vi "Custom Borders to PdfPCells.vi"(0 "PDF Report":T29(xcontrol), 7 "Custom Borders":T11={"Title Row Border"={"Line"={"Thickness"=1.0, "Color"=0}, "Column Borders [ ]"=[]}, "Datas Row Borders [ ]"=[]}, 9 "Cell [ ]":T7[](array[typedef]), 11 "error in (no error)":errorcluster, 12 "Title format":T2={"Font Ref"=refnum, "Leading"=18.0, "Horizontal Aligment"=enum."JUSTIFY", "Vertical Alignment"=enum."BOTTOM"}, 13 "Data Format":T2={"Font Ref"=refnum, "Leading"=18.0, "Horizontal Aligment"=enum."JUSTIFY", "Vertical Alignment"=enum."BOTTOM"}) -> (4 "PDF Report duplicate":T29(xcontrol), 6 "Datas Row Cells [ ]":T1, 10 "Title Row Cells":T6={"Cell Cluster"={"Font Ref"=refnum, "Leading"=18.0, "Horizontal Aligment"=enum."JUSTIFY", "Vertical Alignment"=enum."BOTTOM"}, "PdfPCell [ ]"=[]}, 15 "error out":errorcluster)   [LabVIEW 2012]
doc: "Version 1.0\nDeveloped by Jean-Marc Simard\nCopyright © 2010, Exaprom Inc.\nAll rights reserved.\nLicense: BSD\n\nWith iTextSharp 4.1.6 (http://itextsharp.sourceforge.net)\nunder Mozilla Public License Version 1.1\n(http://www.mozilla.org/MPL/MPL-1.1.html)"
uses:
  Controls/PDF Report Xcontrol/PDF Report.xctl
  Controls/Row Border Title.ctl
  Controls/Cell Border.ctl
  Controls/Row Borders [ ] Datas.ctl
  Controls/Cell Cluster.ctl
  C:/Users/MaxCorp/Documents/TopPerm - Base/DLL/itextsharp.dll
  DLL/itextsharp.dll
  Controls/Font size.ctl
  Controls/Texte alignement.ctl
  Controls/Cell Vertical alignment.ctl
  Controls/Cell Generic Format without Font.ctl
  Controls/Title Cells with refnum.ctl
  Controls/Row PdfPCell [ ] Datas.ctl
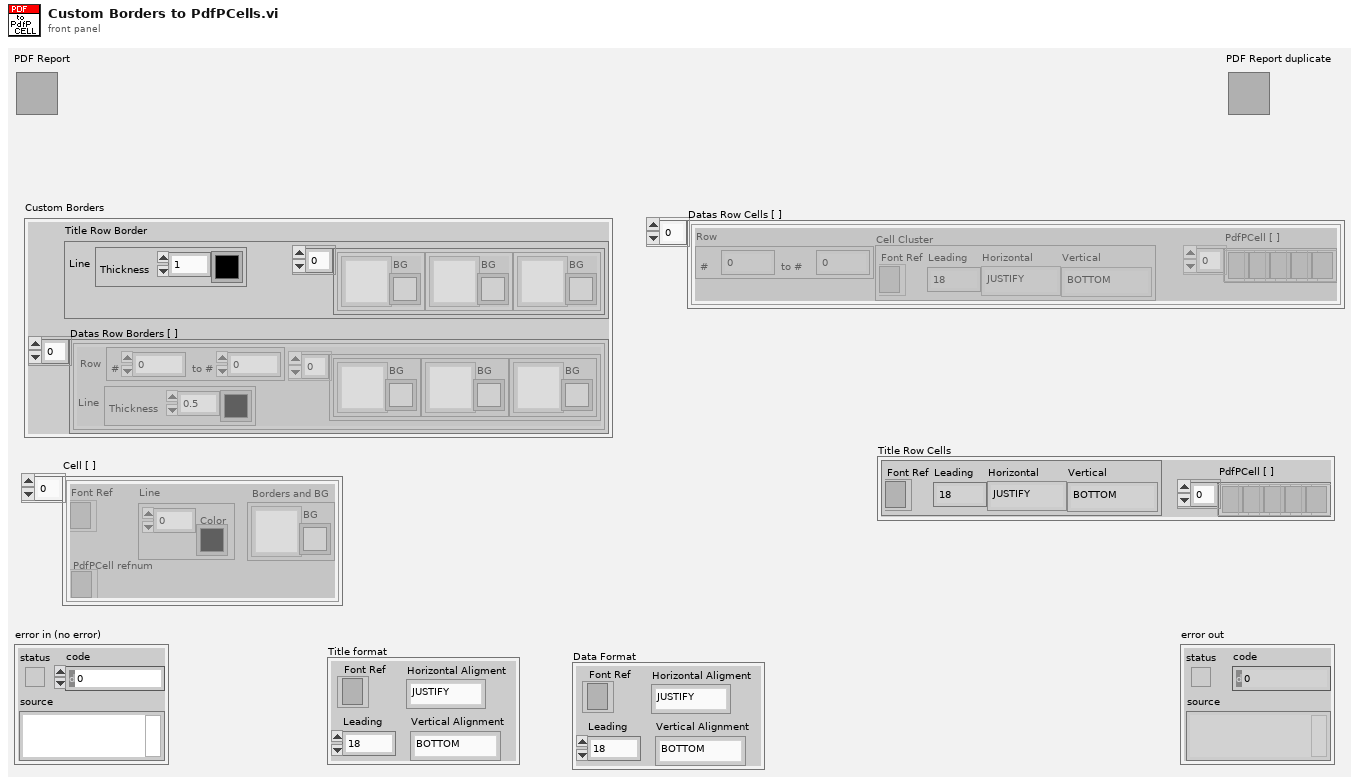
[diagram p1: front panel]
types:
  T1 = typedef "Row PdfPCell [ ] Datas.ctl" = cluster{"Row":cluster{"#":i16, "to #":i16}, "Cell Cluster":T2, "PdfPCell [ ]":refnum<k24>[]}[]
  T2 = typedef "Cell Cluster.ctl" = cluster{"Font Ref":refnum<k24>, "Leading":T3, "Horizontal Aligment":T4, "Vertical Alignment":T5}
  T3 = typedef "Font size.ctl" = sgl
  T4 = typedef "Texte alignement.ctl" = enum16{"Select", "CENTER", "JUSTIFY", "LEFT", "RIGHT"}
  T5 = typedef "Cell Vertical alignment.ctl" = enum16{"TOP", "MIDDLE", "BOTTOM"}
  T6 = typedef "Title Cells with refnum.ctl" = cluster{"Cell Cluster":T2, "PdfPCell [ ]":refnum<k24>[]}
  T7 = typedef "Cell Generic Format without Font.ctl" = cluster{"Font Ref":refnum<k24>, "Line":cluster{"Thickness":sgl, "Color":u32}, "Borders and BG":cluster{"Cell Border":T8, "BG":u32}, "PdfPCell refnum":refnum<k24>}
  T8 = typedef "Cell Border.ctl" = u16
  T9 = typedef "Row Border Title.ctl" = cluster{"Line":cluster{"Thickness":sgl, "Color":u32}, "Column Borders [ ]":cluster{"Cell Border":T8, "BG":u32}[]}
  T10 = typedef "Row Borders [ ] Datas.ctl" = cluster{"Row":cluster{"#":i16, "to #":i16}, "Line":cluster{"Thickness":sgl, "Color":u32}, "Column Borders [ ]":cluster{"Cell Border":T8, "BG":u32}[]}[]
  T11 = cluster{"Title Row Border":T9, "Datas Row Borders [ ]":T10}
  T12 = typedef "Font cluster.ctl" = cluster{"Name":string, "Size":T3, "Color":T13, "Style":cluster{"Bold":bool, "Italic":bool, "Underline":bool, "Strikeout":bool}}
  T13 = typedef "Font color.ctl" = u32
  T14 = typedef "Unit.ctl" = enum16{"inch", "mm"}
  T15 = typedef "Paragraphe cluster.ctl" = cluster{" Aligment":T4, "Line spacing":T16}
  T16 = typedef "Line spacing.ctl" = enum16{"Select", "1.0", "1.5", "2.0"}
  T17 = typedef "Page dimensions.ctl" = cluster{"Start at page":i32, "Orientation":T18, "widht":sgl, "height":sgl, "Margin left":sgl, "Margin right":sgl, "Margin top":sgl, "Margin bottom":sgl}
  T18 = typedef "Page Orientation.ctl" = enum16{"Portrait", "Landscape"}
  T19 = typedef "Image or Table Caption.ctl" = cluster{"Caption":string, "Separator":string, "Position":enum16{"Above", "Below"}}
  T20 = typedef "Header Footer [ ].ctl" = T21[]
  T21 = typedef "Header Footer cluster.ctl" = cluster{"Start page":i32, "Type":T22, "Alignment":T23, "Vertical Alignement":T5, "Image (%)":sgl, "Page #":T24, "Text":string, "Path":string, "Font":T12, "Font refnum":refnum<k24>, "Line":cluster{"Line":T25, "Thickness (points)":sgl, "Colour":T13}}
  T22 = typedef "Header Footer Type.ctl" = enum16{"Select", "Text", "Text + hyperlink", "Page number", "Image", "Image + hyperlink"}
  T23 = typedef "Header footer horiz alignment.ctl" = enum16{"Left", "Center", "Right"}
  T24 = typedef "Page number.ctl" = cluster{"Text 1":string, "Text 2":string, "Text 3":string}
  T25 = typedef "Header Footer Line.ctl" = enum16{"No line", "Horizontal line"}
  T26 = typedef "Watermark cluster2.ctl" = cluster{"Show? (F)":bool, "Type":enum16{"Image", "Text"}, "Opacity (%)":sgl, "Rotate(°)":sgl, "Position":cluster{"Position":T27, "X":sgl, "Y":sgl}, "Image path":path, "Scaled(%)":sgl, "Image refnum":refnum<k24>, "Text":string, "Font":cluster{"Name":string, "Size":T3, "Color":T13}, "Font refnum":refnum<k24>, "Alignment":T23, "Automatic":bool}
  T27 = typedef "Watermark Position.ctl" = enum16{"Absolute", "Center (page)", "Center (text section)"}
  T28 = typedef "System Fonts.ctl" = cluster{"Font name [ ]":string[], "Font and file names [ ]":cluster{"Font name":string, "File name":string}[]}
  T29 = cluster{"Document":refnum<k24>, "Writer":refnum<k24>, "Default Font":refnum<k24>, "Default Font cluster":T12, "Path":path, "Unit (default = mm)":T14, "Paragraphe cluster":T15, "Pages dimensions [ ]":T17[], "Captions":cluster{"Image":T19, "Image counter":u16, "Table":T19, "Table counter":u16, "Font":T12}, "Header":T20, "Footer":T20, "Watermark ":T26, "Actual VI name":string, "System Fonts":T28}
  T30 = cluster{"Row":cluster{"#":i16, "to #":i16}, "Cell Cluster":T2, "PdfPCell [ ]":refnum<k24>[]}
  T31 = cluster{"Row":cluster{"#":i16, "to #":i16}, "Cell Cluster":T2, "PdfPCell [ ]":refnum<k24>[]}[]
  T32 = cluster{"Font Ref":refnum<k24>, "Line":cluster{"Thickness":sgl, "Color":u32}, "Borders and BG":cluster{"Cell Border":T8, "BG":u32}}
  T33 = cluster{"Font Ref":refnum<k24>, "Line":cluster{"Thickness":sgl, "Color":u32}, "Cluster 2":cluster{"Cell Border":T8, "BG":u32}}
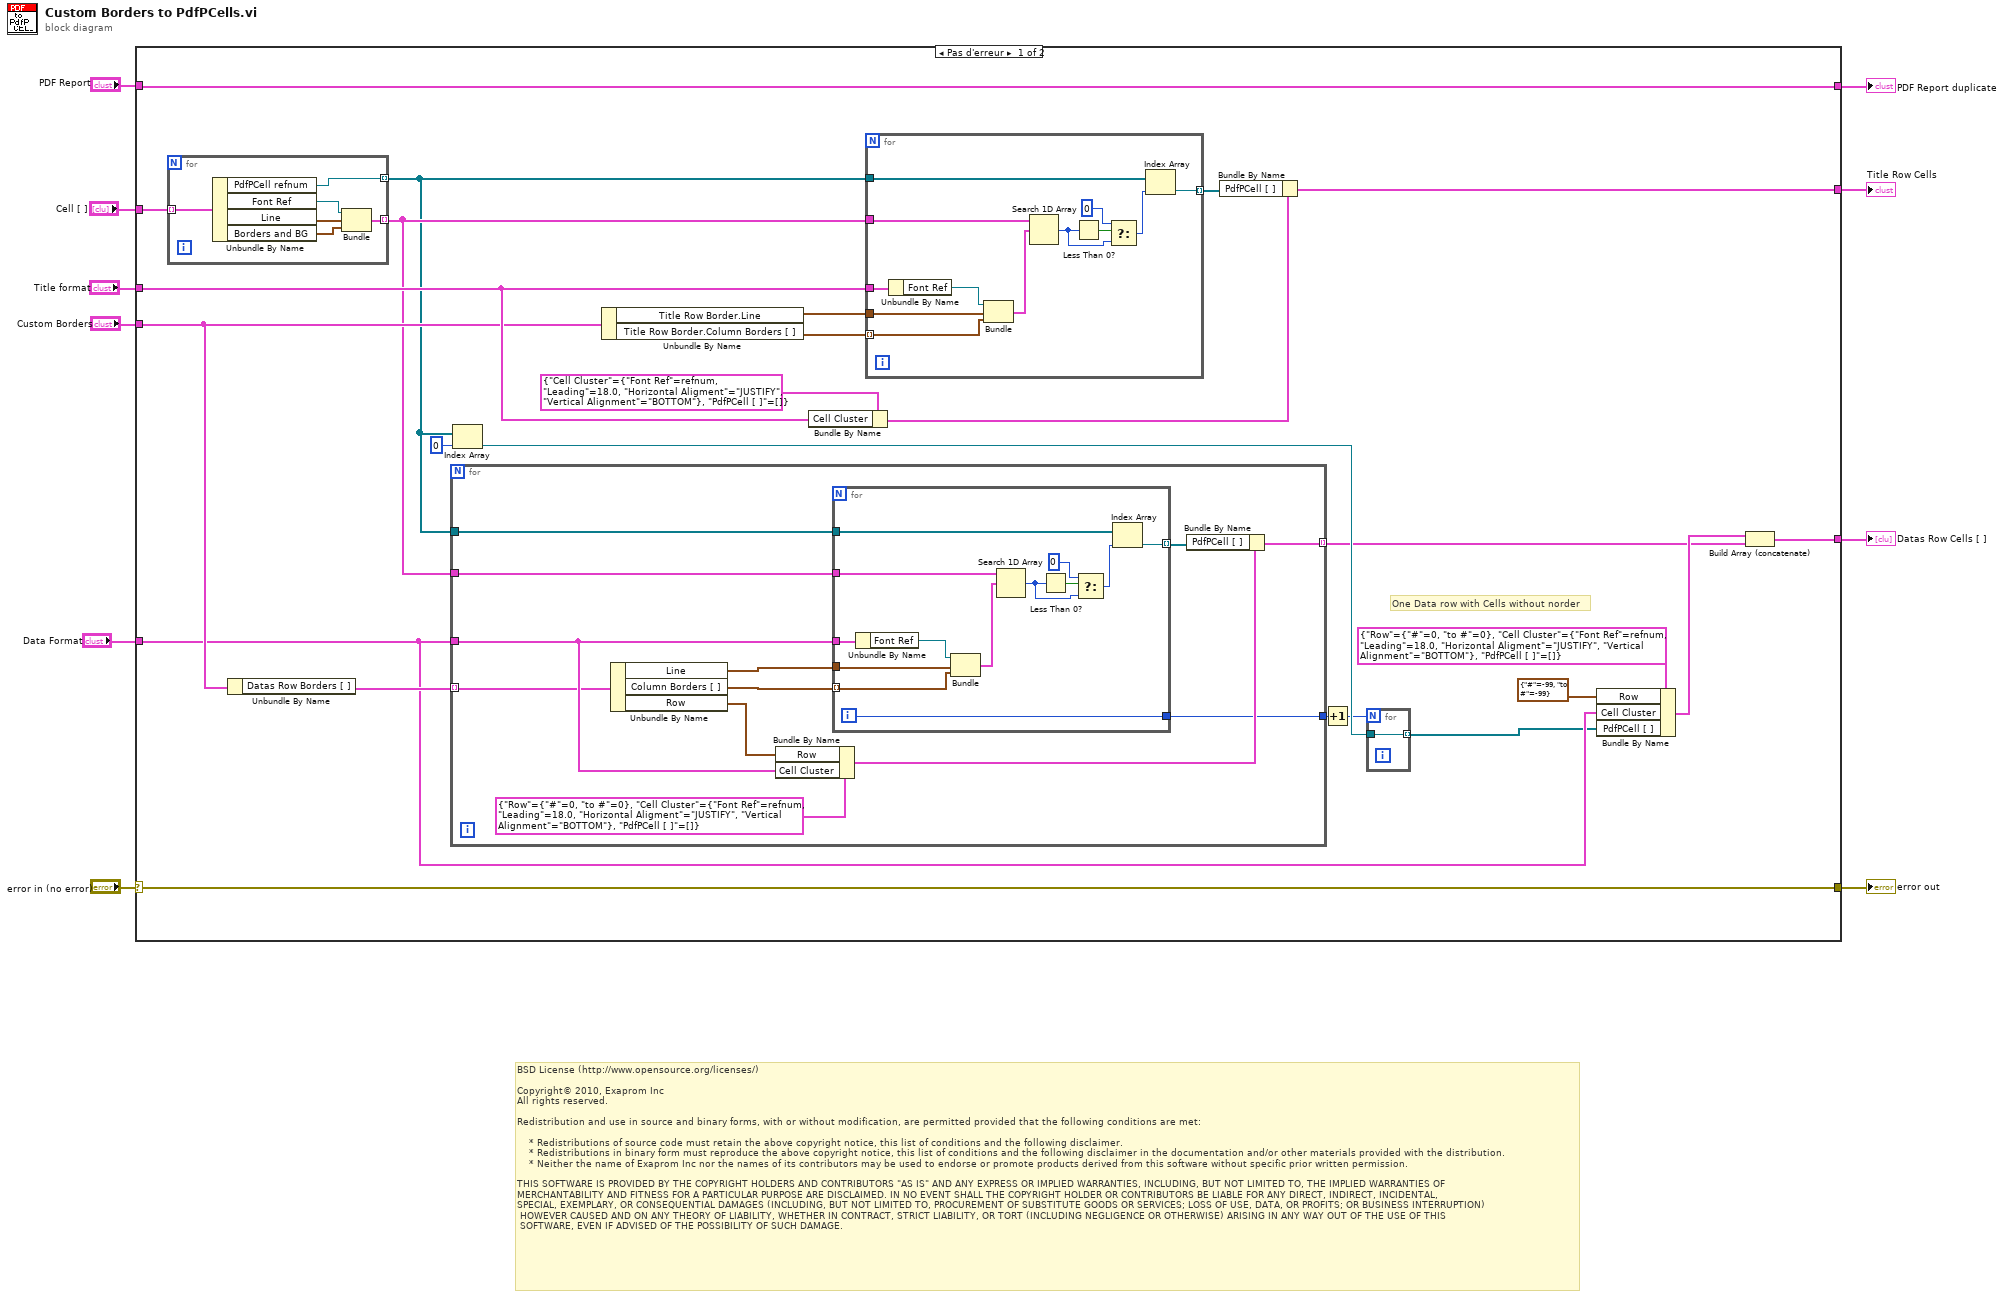
[diagram p0: block diagram]
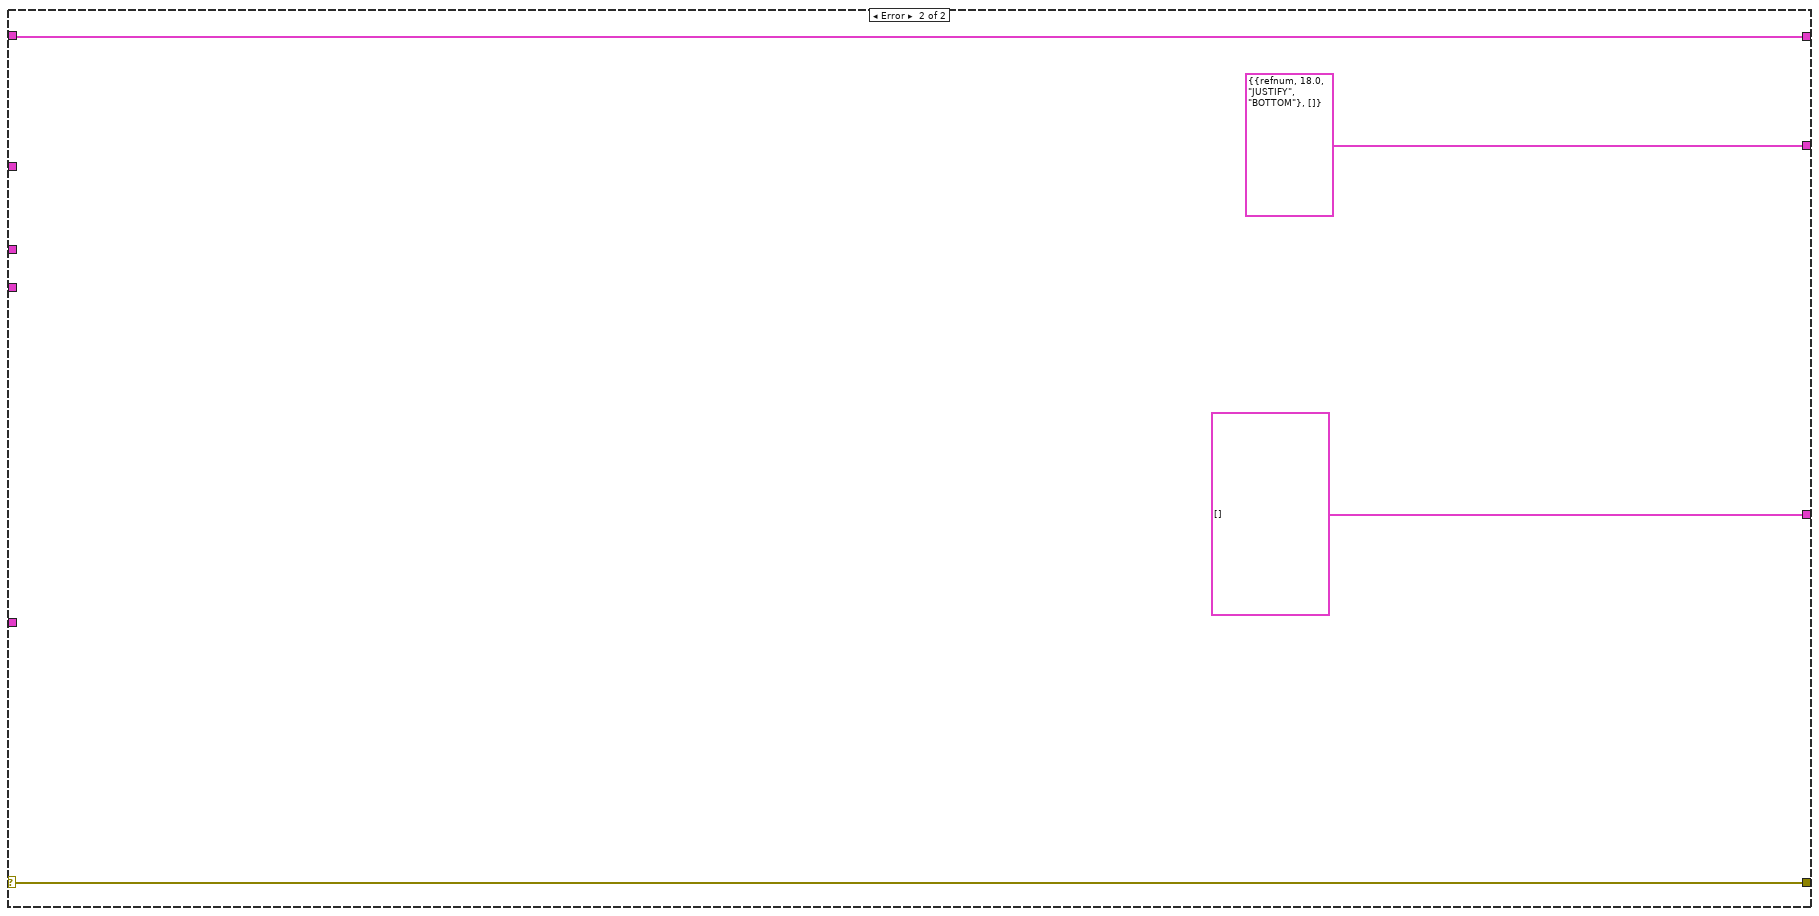
[diagram p2: hidden frame]
diagram:
  # "BSD License (http://www.opensource.org/licenses/)\n\nCopyright© 2010, Exaprom Inc\nAll rights reserved.\n\nRedistribution and use in source and binary forms, with or without modification, are permitted provided that the following conditions are met:\n\n    * Redistributions of source code must retain the above copyright notice, this list of conditions and the following disclaimer.\n    * Redistributions in binary form must reproduce the above copyright notice, this list of conditions and the following disclaimer in the documentation and/or other materials provided with the distribution.\n    * Neither the name of Exaprom Inc nor the names of its contributors may be used to endorse or promote products derived from this software without specific prior written permission.\n\nTHIS SOFTWARE IS PROVIDED BY THE COPYRIGHT HOLDERS AND CONTRIBUTORS \"AS IS\" AND ANY EXPRESS OR IMPLIED WARRANTIES, INCLUDING, BUT NOT LIMITED TO, THE IMPLIED WARRANTIES OF \nMERCHANTABILITY AND FITNESS FOR A PARTICULAR PURPOSE ARE DISCLAIMED. IN NO EVENT SHALL THE COPYRIGHT HOLDER OR CONTRIBUTORS BE LIABLE FOR ANY DIRECT, INDIRECT, INCIDENTAL,\nSPECIAL, EXEMPLARY, OR CONSEQUENTIAL DAMAGES (INCLUDING, BUT NOT LIMITED TO, PROCUREMENT OF SUBSTITUTE GOODS OR SERVICES; LOSS OF USE, DATA, OR PROFITS; OR BUSINESS INTERRUPTION)\n HOWEVER CAUSED AND ON ANY THEORY OF LIABILITY, WHETHER IN CONTRACT, STRICT LIABILITY, OR TORT (INCLUDING NEGLIGENCE OR OTHERWISE) ARISING IN ANY WAY OUT OF THE USE OF THIS\n SOFTWARE, EVEN IF ADVISED OF THE POSSIBILITY OF SUCH DAMAGE."
  n1 = case shown="Pas d'erreur" "error in (no error)" {
    selector: "error in (no error)" -> [w12 w82]
    tunnel: "PDF Report" -> [w35 w83]
    tunnel: [w35 w83] -> w10
    tunnel: [w12 w82] -> w1
    tunnel: "Custom Borders" -> [w26 _]
    tunnel: "Cell [ ]" -> [w33 _]
    tunnel: "Title format" -> [w30 _]
    tunnel: [w27 T6 {"Cell Cluster"={"Font Ref"=refnum, "Leading"=18.0, "Horizontal Aligment"=enum."JUSTIFY", "Vertical Alignment"=enum."BOTTOM"}, "PdfPCell [ ]"=[]} ("Title Row Cells")] -> w4
    tunnel: "Data Format" -> [w17 _]
    tunnel: [w13 T31 []] -> w2
    frame No Error {
      # "One Data row with Cells without norder"
      n2 = for {
        tunnel: w33 -> [w67] mode=indexing
        tunnel: [w63] -> w25 mode=indexing
        tunnel: [w62] -> w22 mode=indexing
        n3 = Unbundle By Name(w67) -> ("PdfPCell refnum"=w62:refnum<k24>, "Font Ref"=w65:refnum<k24>, "Line"=w66:cluster{"Thickness":sgl, "Color":u32}, "Borders and BG"=w64:cluster{"Cell Border":T8, "BG":u32})
        n4 = Bundle("Font Ref"=w65, "Line"=w66, "Borders and BG"=w64) -> (w63:T32)  [unwired: 1 out]
      }
      n5 = Unbundle By Name(w26) -> ("Datas Row Borders [ ]"=w24:T10)
      n6 = for {
        tunnel: w25 -> [w44]
        tunnel: w22 -> [w43]
        tunnel: w17 -> [w42]
        tunnel: w24 -> [w41] mode=indexing
        tunnel: [w39] -> w14 mode=indexing
        tunnel: [w38] -> w23
        n7 = Unbundle By Name(w41) -> ("Line"=w46:cluster{"Thickness":sgl, "Color":u32}, "Column Borders [ ]"=w45:cluster{"Cell Border":T8, "BG":u32}[], "Row"=w40:cluster{"#":i16, "to #":i16})
        n8 = Bundle By Name(cluster=T30 {"Row"={"#"=0, "to #"=0}, "Cell Cluster"={"Font Ref"=refnum, "Leading"=18.0, "Horizontal Aligment"=enum."JUSTIFY", "Vertical Alignment"=enum."BOTTOM"}, "PdfPCell [ ]"=[]} ("Row Borders with refnum"), "Row"=w40, "Cell Cluster"=w42) -> (w47:T30)
        n9 = for {
          tunnel: w45 -> [w59] mode=indexing
          tunnel: w44 -> [w57]
          tunnel: w42 -> [w61]
          tunnel: w46 -> [w60]
          tunnel: w43 -> [w55]
          tunnel: [w50] -> w48 mode=indexing
          tunnel: [w49] -> w38
          i -> [w49]
          n10 = Unbundle By Name(w61) -> ("Font Ref"=w58:refnum<k24>)
          n11 = Bundle("Font Ref"=w58, "Line"=w60, "Cluster 2"=w59) -> (w56:T33)  [unwired: 1 out]
          n12 = Search 1D Array(1D array=w57, element=w56) -> (index of element=w53:i32)  [unwired: 1 out]
          n13 = Less Than 0?(x=w53) -> (x < 0?=w54:bool)
          n14 = Select(t=0, s=w54, f=w53) -> (s? t:f=w52:i32)
          n15 = Index Array(array=w55, index=w52) -> (element=w50:refnum<k24>)
        }
        n16 = Bundle By Name(cluster=w47, "PdfPCell [ ]"=w48) -> (w39:T30)
      }
      n17 = Index Array(array=w22, index=0) -> (element=w20:refnum<k24>)
      n18 = Unbundle By Name(w26) -> ("Title Row Border.Line"=w32:cluster{"Thickness":sgl, "Color":u32}, "Title Row Border.Column Borders [ ]"=w34:cluster{"Cell Border":T8, "BG":u32}[])
      n19 = Bundle By Name(cluster=T6 {"Cell Cluster"={"Font Ref"=refnum, "Leading"=18.0, "Horizontal Aligment"=enum."JUSTIFY", "Vertical Alignment"=enum."BOTTOM"}, "PdfPCell [ ]"=[]} ("Title Row Cells"), "Cell Cluster"=w30) -> (w29:T6)
      n20 = for {
        tunnel: w34 -> [w77] mode=indexing
        tunnel: w25 -> [w75]
        tunnel: w30 -> [w79]
        tunnel: w32 -> [w78]
        tunnel: w22 -> [w73]
        tunnel: [w68] -> w28 mode=indexing
        n21 = Unbundle By Name(w79) -> ("Font Ref"=w76:refnum<k24>)
        n22 = Bundle("Font Ref"=w76, "Line"=w78, "Cluster 2"=w77) -> (w74:T33)  [unwired: 1 out]
        n23 = Search 1D Array(1D array=w75, element=w74) -> (index of element=w71:i32)  [unwired: 1 out]
        n24 = Less Than 0?(x=w71) -> (x < 0?=w72:bool)
        n25 = Select(t=0, s=w72, f=w71) -> (s? t:f=w70:i32)
        n26 = Index Array(array=w73, index=w70) -> (element=w68:refnum<k24>)
      }
      n27 = Bundle By Name(cluster=w29, "PdfPCell [ ]"=w28) -> (w27:T6)
      n28 = Increment(x=w23) -> (x+1=w11:i32)
      n29 = for {
        N: w11 -> [_]
        tunnel: w20 -> [w36]
        tunnel: [w36] -> w16 mode=indexing
      }
      n30 = Bundle By Name(cluster=T30 {"Row"={"#"=0, "to #"=0}, "Cell Cluster"={"Font Ref"=refnum, "Leading"=18.0, "Horizontal Aligment"=enum."JUSTIFY", "Vertical Alignment"=enum."BOTTOM"}, "PdfPCell [ ]"=[]} ("Row Borders with refnum"), "Row"=cluster{"#":i16, "to #":i16} {"#"=-99, "to #"=-99}, "Cell Cluster"=w17, "PdfPCell [ ]"=w16) -> (w15:T30)
      n31 = Build Array (concatenate)(w15, w14) -> (w13:T31)
    }
    frame Error {
    }
  }
  "PDF Report duplicate" <- w10
  "error out" <- w1
  "Title Row Cells" <- w4
  "Datas Row Cells [ ]" <- w2
